vi "Initial.vi"(8 "error in (no error)":errorcluster, 10 "Project name":string="Demo") -> (0 "error out":errorcluster, 3 "Return":i32)   [LabVIEW 2015]
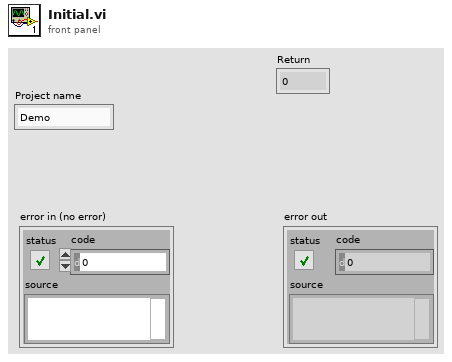
[diagram p1: front panel]
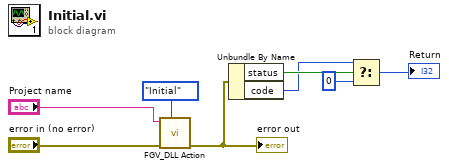
[diagram p0: block diagram]
diagram:
  n1 = call "FGV_DLL Action.vi"("State"=enum16{"Initial", "Run", "Close"}."Initial", "Error In"="error in (no error)", "Project name"="Project name") -> ("Error Out"=w2:errorcluster)  [unwired: 8 in]
  "error out" <- w2
  n2 = Unbundle By Name(w2) -> ("status"=w6:bool, "code"=w5:i32)
  n3 = Select(t=w5, s=w6, f=0) -> (s? t:f=→"Return":i32)
